vi "getInterpolationCoefficients.vi"(11 "Deflection to energy calibration file":path) -> (2 "piecewise polynomial":T1 {"x locations" format="%.4g"; "coefficients" format="%.4g"}, 3 "path out":path)   [LabVIEW 2014]
uses:
  <vilib>/gmath/interp.llb/in_piecewise interp poly control.ctl
  <vilib>/Utility/file.llb/Read From Spreadsheet File (DBL).vi
  <vilib>/gmath/NI_Gmath.lvlib
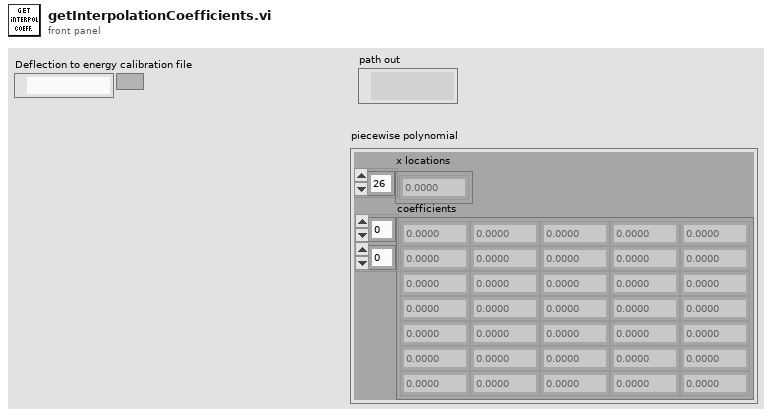
[diagram p1: front panel]
types:
  T1 = typedef "NI_Gmath.lvlib/in_piecewise interp poly control.ctl" = cluster{"x locations":dbl[], "coefficients":dbl[][]}
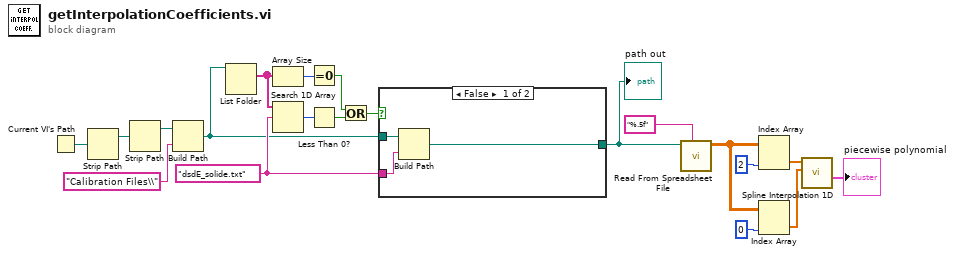
[diagram p0: block diagram]
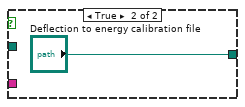
[diagram p2: hidden frame]
diagram:
  w12 = "dsdE_solide.txt" ("element")
  n1 = Current VI's Path() -> (path=w19:path)
  n2 = Strip Path(path=w19) -> (stripped path=w20:path)  [unwired: 1 out]
  n3 = Strip Path(path=w20) -> (stripped path=w1:path)  [unwired: 1 out]
  n4 = Build Path(base path=w1, name or relative path="Calibration Files\\") -> (appended path=w3:path)
  n5 = List Folder(path=w3) -> (filenames=w2:string[])  [unwired: 3 in, 3 out]
  n6 = Array Size(array=w2) -> (size(s)=w17:i32)
  n7 = Search 1D Array(1D array=w2, element=w12) -> (index of element=w16:i32)  [unwired: 1 in]
  n8 = Equal To 0?(x=w17) -> (x = 0?=w15:bool)
  n9 = Less Than 0?(x=w16) -> (x < 0?=w14:bool)
  n10 = Or(x=w15, y=w14) -> (x .or. y?=w13:bool)
  n11 = case shown="False" w13 {
    tunnel: w3 -> [w23 _]
    tunnel: w12 -> [w22 _]
    tunnel: [w21 "Deflection to energy calibration file"] -> w11
    frame False {
      n12 = Build Path(base path=w23, name or relative path=w22) -> (appended path=w21:path)
    }
    frame True {
    }
  }
  "path out" <- w11
  n13 = call-poly <vilib>:"Read From Spreadsheet File.vi"("format (%.3f)"="%.5f", "file path (dialog if empty)"=w11) -> ("all rows"=w9:dbl[][])  [unwired: 5 in, 4 out]
  n14 = Index Array(array=w9, index (col)=2 ("disabled index (col)")) -> (element=w6:dbl[])  [unwired: 1 in]
  n15 = Index Array(array=w9, index (col)=0 ("disabled index (col)")) -> (element=w5:dbl[])  [unwired: 1 in]
  n16 = call <vilib>:"Spline Interpolation 1D.vi"("X"=w5, "Y"=w6) -> ("piecewise polynomial"=→"piecewise polynomial":T1)  [unwired: 7 in, 2 out]
